vi "AssertCellValue.vi"(0 "VI Reference In":refnum<vi>, 1 "Test Label":string, 2 "delimiter (>>)":string=">>", 3 "Assert Only? (F)":bool, 5 "Control Path":string, 7 "Row Index":i32, 9 "Item Value":string, 11 "Error In":errorcluster, 12 "Assert Interval(10 ms)":u32=10, 13 "Timeout(5 sec)":dbl=5.0, 14 "Column Index":i32) -> (4 "VI Reference Out":refnum<vi>, 6 "Asserted Value":string, 15 "Error Out":errorcluster)   [LabVIEW 2016, in "Drona.lvlib" / "AssertControlValue.lvlib" / "AssertTable.lvlib"]
doc: "Asserts if the item on specified index in the Table is equal.\n\nThe input control name is given as a string, incase of the path, use delimiters in between the path.\nThis VI gets the control value until the value is equal to the input value."
uses:
  AssertTable.lvlib
  Get/GetControlRef/GetControlRefByPath.vi
  <vilib>/Utility/error.llb/Error Cluster From Error Code.vi
  <vilib>/addons/_JKI Toolkits/Caraya/classes/Assert/Assert Equal Value_Variant.vi
  <vilib>/ErrorRing/Error Ring.xnode
  <vilib>/addons/_JKI Toolkits/Caraya/classes/Assert/Assert.lvclass
  Get/GetControlRef/GetControlRef.lvlib
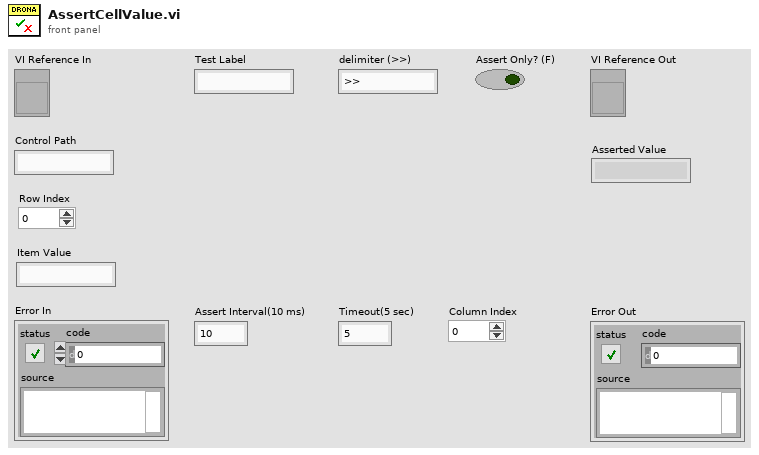
[diagram p1: front panel]
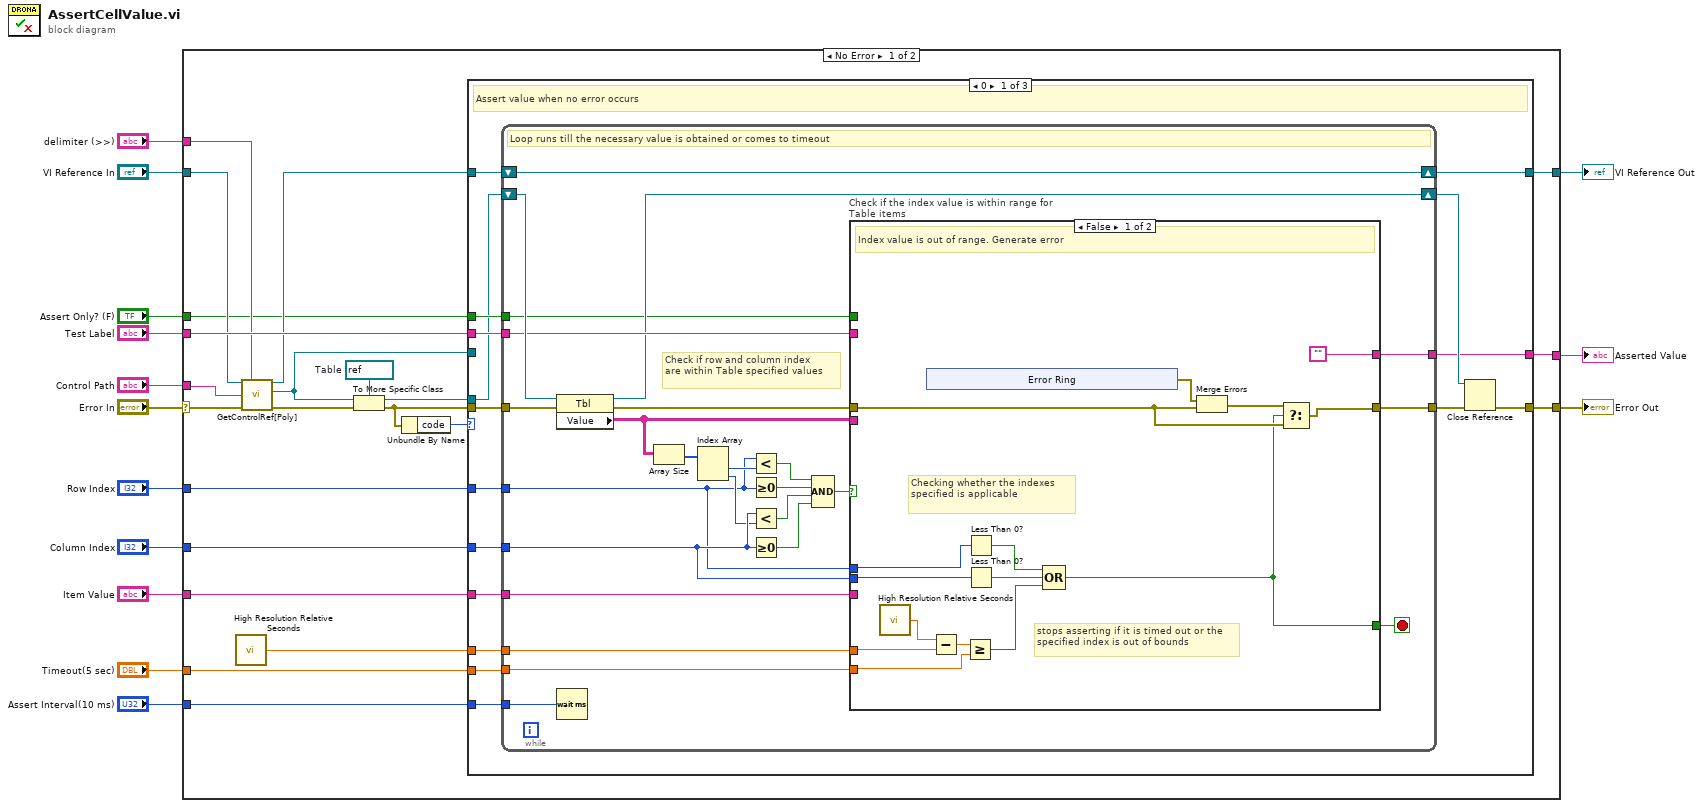
[diagram p0: block diagram]
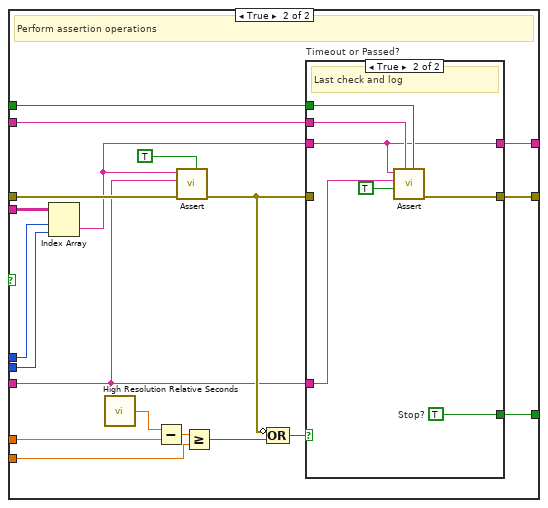
[diagram p2: hidden frame]
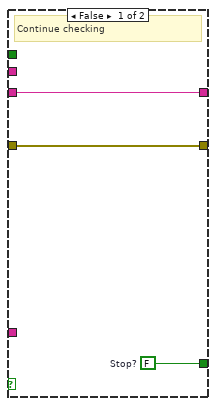
[diagram p3: hidden frame]
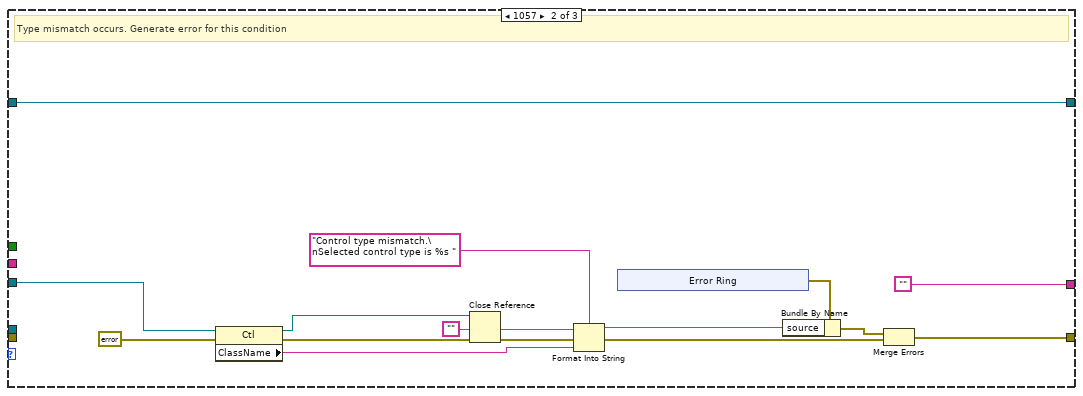
[diagram p4: hidden frame]
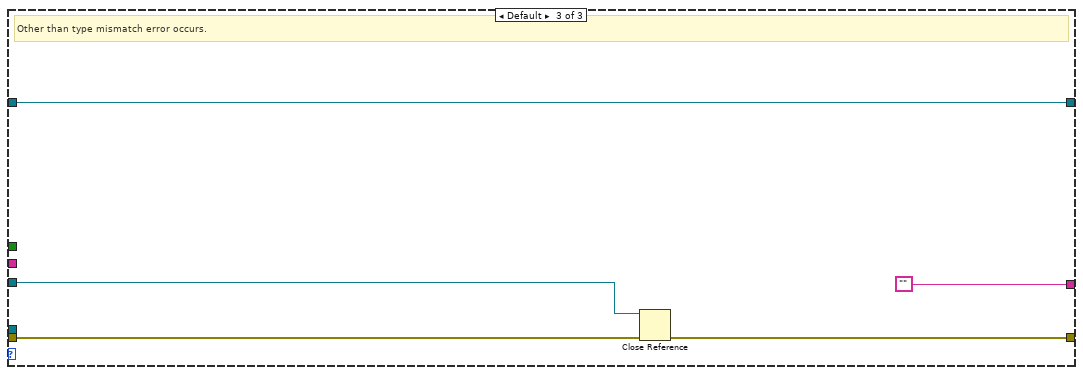
[diagram p5: hidden frame]
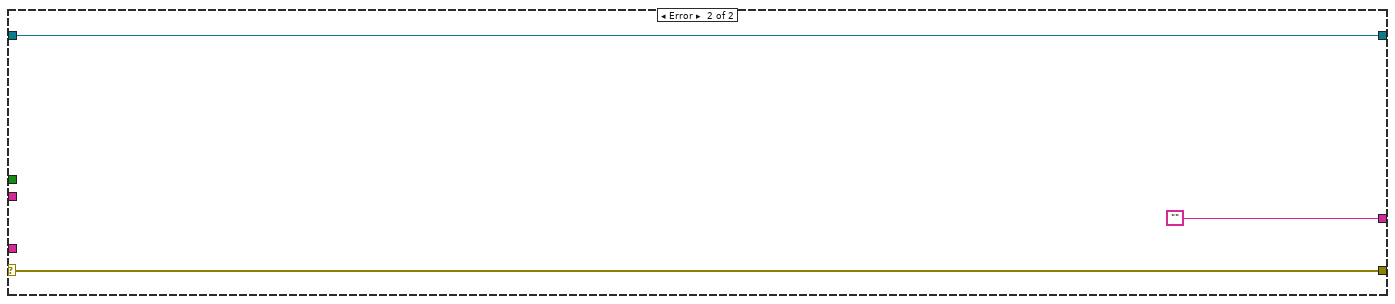
[diagram p6: hidden frame]
diagram:
  n1 = case shown="No Error" "Error In" {
    selector: "Error In" -> [w31 w154]
    tunnel: "Timeout(5 sec)" -> [w36 _]
    tunnel: [w35 w153] -> w13
    tunnel: "Row Index" -> [w34 _]
    tunnel: [w25 w154] -> w12
    tunnel: "Assert Interval(10 ms)" -> [w33 _]
    tunnel: "Test Label" -> [w32 _]
    tunnel: "VI Reference In" -> [w30 w153]
    tunnel: "Control Path" -> [w29 _]
    tunnel: "delimiter (>>)" -> [w24 _]
    tunnel: "Assert Only? (F)" -> [w23 _]
    tunnel: [w22 ""] -> w2
    tunnel: "Item Value" -> [w19 _]
    tunnel: "Column Index" -> [w15 _]
    frame No Error {
      w21 = refnum<vi> refnum  # Table
      n2 = call <vilib>:"High Resolution Relative Seconds.vi"() -> ("relative seconds"=w28:dbl)
      n3 = call-poly "GetControlRef[Poly].vi"("VI Reference In"=w30, "delimiter (>>)"=w24, "Control Path"=w29, "error In"=w31) -> ("VI Reference Out"=w26:refnum<vi>, "Ctl Refnum"=w16:refnum<vi>, "error out"=w27:errorcluster)  [unwired: 9 in]
      n4 = To More Specific Class(target class=w21, reference=w16, error in=w27) -> (specific class reference=w20:refnum<vi>, error out=w18:errorcluster)
      n5 = Unbundle By Name(w18) -> ("code"=w17:i32)
      n6 = case shown="0" w17 {
        tunnel: w36 -> [w52 _ _]
        tunnel: [w51 w140 w151] -> w35
        tunnel: w34 -> [w50 _ _]
        tunnel: w33 -> [w48 _ _]
        tunnel: w32 -> [w47 _ _]
        tunnel: w28 -> [w46 _ _]
        tunnel: w26 -> [w45 w140 w151]
        tunnel: [w44 w128 w148] -> w25
        tunnel: w23 -> [w42 _ _]
        tunnel: [w41 "" ""] -> w22
        tunnel: w18 -> [w40 _ w150]
        tunnel: w20 -> [w39 _ _]
        tunnel: w19 -> [w38 _ _]
        tunnel: w16 -> [_ w127 w147]
        tunnel: w15 -> [w37 _ _]
        frame 0 {
          # "Assert value when no error occurs"
          n7 = while {
            tunnel: w50 -> [w53]
            tunnel: w52 -> [w76]
            tunnel: w46 -> [w77]
            tunnel: w40 -> [w71]
            tunnel: [w74] -> w49
            tunnel: w48 -> [w72]
            tunnel: w47 -> [w68]
            shift-right: [w69] -> w51
            shift-left: w45 -> [w69]
            shift-right: [w67] -> w43
            shift-left: w39 -> [w70]
            tunnel: w42 -> [w66]
            tunnel: [w65] -> w41
            tunnel: w38 -> [w64]
            tunnel: w37 -> [w58]
            stop <- w75 stop-if-true
            # "Check if row and column index \nare within Table specified values"
            # "Loop runs till the necessary value is obtained or comes to timeout"
            n8 = property on="Property Node" class="Tbl"(reference=w70, error in=w71) -> (reference out=w67:refnum<vi>, error out=w73:errorcluster, "Value"=w57:string[][])
            n9 = Wait (ms)(milliseconds to wait=w72) -> ()  [unwired: 1 out]
            n10 = Array Size(array=w57) -> (size(s)=w56:i32[])
            n11 = Index Array(array=w56) -> (element #1=w55:i32, element #2=w54:i32)  [unwired: 2 in]
            n12 = Less?(x=w53, y=w55) -> (x < y?=w63:bool)
            n13 = Greater Or Equal To 0?(x=w53) -> (x >= 0?=w62:bool)
            n14 = Less?(x=w58, y=w54) -> (x < y?=w61:bool)
            n15 = Greater Or Equal To 0?(x=w58) -> (x >= 0?=w60:bool)
            n16 = Compound Arithmetic op=AND(w63, w62, w61, w60) -> (w59:bool)
            n17 = case "Check if the index value is within range for Table items" shown="False" w59 {
              tunnel: w77 -> [w81 w116]
              tunnel: w76 -> [w80 w113]
              tunnel: [w78 w105] -> w75
              tunnel: [w79 w106] -> w74
              tunnel: w68 -> [_ w111]
              tunnel: w66 -> [_ w104]
              tunnel: ["" w103] -> w65
              tunnel: w64 -> [_ w102]
              tunnel: w57 -> [_ w101]
              tunnel: w73 -> [w84 w112]
              tunnel: w58 -> [w82 w99]
              tunnel: w53 -> [w83 w98]
              frame False {
                # "stops asserting if it is timed out or the specified index is out of bounds"
                # "Checking whether the indexes specified is applicable"
                # "Index value is out of range. Generate error"
                n18 = call <vilib>:"High Resolution Relative Seconds.vi"() -> ("relative seconds"=w89:dbl)
                n19 = xnode "Error Ring"() -> ("error out"=w91:errorcluster)
                n20 = Subtract(x=w89, y=w81) -> (x-y=w90:dbl)
                n21 = Greater Or Equal?(x=w90, y=w80) -> (x >= y?=w88:bool)
                n22 = Less Than 0?(x=w83) -> (x < 0?=w86:bool)
                n23 = Less Than 0?(x=w82) -> (x < 0?=w87:bool)
                n24 = Compound Arithmetic op=OR(w86, w87, w88) -> (w78:bool)
                n25 = Merge Errors(w91, w84) -> (w85:errorcluster)
                n26 = Select(t=w85, s=w78, f=w84) -> (s? t:f=w79:errorcluster)
              }
              frame True {
                # "Perform assertion operations"
                n27 = Index Array(array=w101, index (row)=w98, index (col)=w99) -> (element=w100:string)
                n28 = call <vilib>:"High Resolution Relative Seconds.vi"() -> ("relative seconds"=w115:dbl)
                n29 = Subtract(x=w115, y=w116) -> (x-y=w114:dbl)
                n30 = call-poly <vilib>:"Assert.vi"("Assert Only? (F)"=TRUE, "error in (no error)"=w112, "Y"=w102, "X"=w100) -> ("error out"=w109:errorcluster)  [unwired: 6 in, 1 out]
                n31 = Greater Or Equal?(x=w114, y=w113) -> (x >= y?=w110:bool)
                n32 = Compound Arithmetic op=OR(invert w109, w110) -> (w108:bool)
                n33 = case "Timeout or Passed?" shown="True" w108 {
                  tunnel: w109 -> [w119 _]
                  tunnel: w102 -> [_ w125]
                  tunnel: w100 -> [w117 w120]
                  tunnel: w111 -> [_ w126]
                  tunnel: [w119 w124] -> w106
                  tunnel: [w118 w123] -> w105
                  tunnel: w104 -> [_ w121]
                  tunnel: [w117 w120] -> w103
                  frame False {
                    w118 = FALSE  # Stop?
                    # "Continue checking"
                  }
                  frame True {
                    w123 = TRUE  # Stop?
                    # "Last check and log"
                    n34 = call-poly <vilib>:"Assert.vi"("Assert Only? (F)"=w121, "Label"=w126, "Register with caller test (F)"=TRUE, "Y"=w125, "X"=w120) -> ("error out"=w124:errorcluster)  [unwired: 5 in, 1 out]
                  }
                }
              }
            }
          }
          n35 = Close Reference(reference=w43, error in (no error)=w49) -> (error out=w44:errorcluster)
        }
        frame 1057 {
          # "Type mismatch occurs. Generate error for this condition"
          n36 = property class="Ctl"(reference=w127, error in=errorcluster {"status"=FALSE, "code"=0, "source"=""} ("error out")) -> (reference out=w129:refnum<vi>, error out=w139:errorcluster, "ClassName"=w136:string)
          n37 = Close Reference(reference=w129, error in (no error)=w139) -> (error out=w130:errorcluster)
          n38 = Format Into String(format string="Control type mismatch.\nSelected control type is %s ", initial string="", error in=w130, w136) -> (resulting string=w133:string, error out=w131:errorcluster)
          n39 = xnode "Error Ring"() -> ("error out"=w134:errorcluster)
          n40 = Bundle By Name(cluster=w134, "source"=w133) -> (w132:errorcluster)
          n41 = Merge Errors(w132, w131) -> (w128:errorcluster)
        }
        frame Default {
          # "Other than type mismatch error occurs."
          n42 = Close Reference(reference=w147, error in (no error)=w150) -> (error out=w148:errorcluster)
        }
      }
    }
    frame Error {
    }
  }
  "Error Out" <- w12
  "VI Reference Out" <- w13
  "Asserted Value" <- w2
